vi "CSM - Read Config Cluster(Variant).vi"(4 "Write If not found?":bool, 5 "Section Name(\"\" as Default)":string, 7 "error in (no error)":errorcluster, 9 "Variant":variant) -> (1 "error out":errorcluster, 3 "Variant":variant)   [LabVIEW 2017, in "INI-Static-Variable-Support.lvlib"]
uses:
  INI-Static-Variable-Support.lvlib
  _fgv-oper.ctl
  fda69cd8-9796-4e90-9db0-f860da454eb2.vi
  global-csm-ini-db-change-flag.vi
  <userlib>/_NEVSTOP/Communicable State Machine(CSM)/addons/API-String-Arugments-Support/_Support/Data To API String Arguments.vi
  <userlib>/_NEVSTOP/Communicable State Machine(CSM)/addons/API-String-Arugments-Support/API String Arguments Support.lvlib
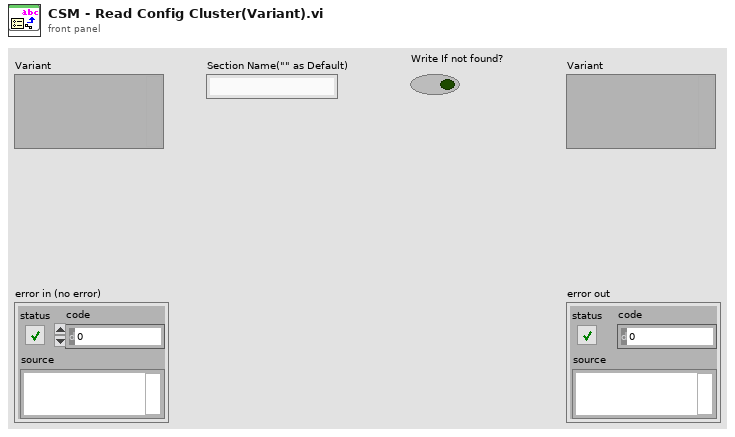
[diagram p1: front panel]
types:
  T1 = typedef "INI-Static-Variable-Support.lvlib/_fgv-oper.ctl" = enum16{"Read", "Write", "Sync"}
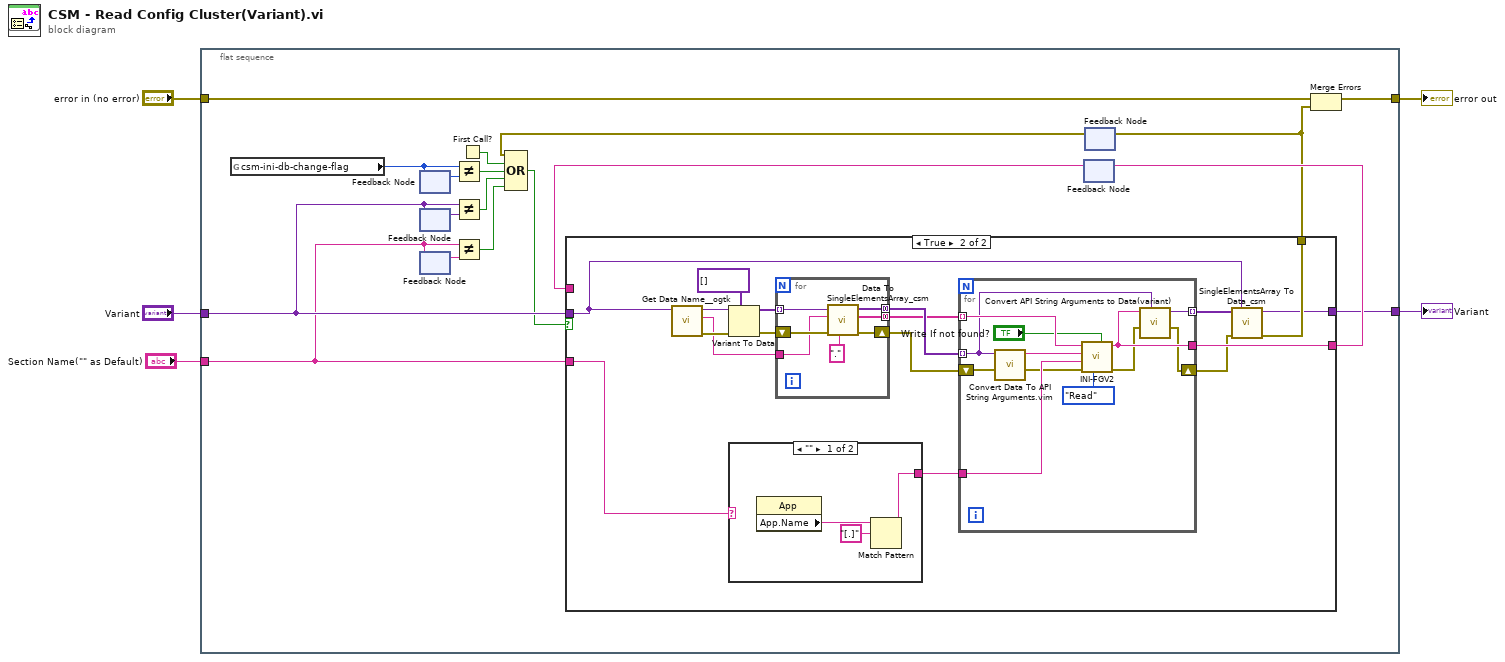
[diagram p0: block diagram]
diagram:
  n1 = flat-sequence {
    tunnel: [w23] -> w5
    tunnel: "error in (no error)" -> [w22]
    tunnel: "Variant" -> [w15]
    tunnel: "Section Name(\"\" as Default)" -> [w14]
    tunnel: [w6] -> w1
    frame #0 {
      n2 = global read "global-csm-ini-db-change-flag.vi" "csm-ini-db-change-flag"() -> (w21:u32)
      n3 = feedback #1() -> (w20:u32)  [unwired: 1 in]
      n4 = feedback-in #1(w21) -> ()
      n5 = feedback #2() -> (w17:variant)  [unwired: 1 in]
      n6 = feedback-in #2(w15) -> ()
      n7 = feedback #3() -> (w16:string)  [unwired: 1 in]
      n8 = feedback-in #3(w14) -> ()
      n9 = Not Equal?(x=w21, y=w20) -> (x != y?=w19:bool)
      n10 = Not Equal?(x=w15, y=w17) -> (x != y?=w13:bool)
      n11 = Not Equal?(x=w14, y=w16) -> (x != y?=w12:bool)
      n12 = First Call?() -> (First Call?: T/F=w18:bool)
      n13 = feedback #4() -> (w10:string)  [unwired: 1 in]
      n14 = feedback #5() -> (w8:errorcluster)  [unwired: 1 in]
      n15 = Compound Arithmetic op=OR(w8, w18, w19, w13, w12) -> (w7:bool)
      n16 = case shown="True" w7 {
        tunnel: [_ w35] -> w9
        tunnel: [w25 w42] -> w11
        tunnel: w15 -> [w24 w31]
        tunnel: w14 -> [_ w41]
        tunnel: w10 -> [w25 _]
        tunnel: [w24 w34] -> w6
        frame False {
        }
        frame True {
          n17 = call <userlib>:"Get Data Name__ogtk.vi"("Data"=w31) -> ("error out"=w27:errorcluster, "Data Name"=w26:string, "Data dup"=w28:variant)  [unwired: 8 in]
          n18 = Variant To Data(error in=w27, type=variant[] [] ("Array"), Variant=w28) -> (data=w30:variant[], error out=w29:errorcluster)
          n19 = case shown="\"\"" w41 {
            selector: w41 -> [_ w65]
            tunnel: [w62 w65] -> w40
            frame "" {
              n20 = property class="App"() -> ("App.Name"=w63:string)  [unwired: 2 in, 2 out]
              n21 = Match Pattern(string=w63, regular expression="[.]") -> (before substring=w62:string)  [unwired: 1 in, 3 out]
            }
            frame Default {
            }
          }
          n22 = for {
            tunnel: [w48] -> w39 mode=concatenating
            tunnel: [w47] -> w38 mode=concatenating
            tunnel: w30 -> [w45] mode=indexing
            shift-right: [w46] -> w33
            shift-left: w29 -> [w44]
            tunnel: w26 -> [w43]
            n23 = call <userlib>:"Data To SingleElementsArray_csm.vi"("Seperator(/)"=".", "error in (no error)"=w44, "parentUrl"=w43, "Cluster"=w45) -> ("error out"=w46:errorcluster, "Full NameList"=w47:string[], "DataElementArray"=w48:variant[])  [unwired: 5 in]
          }
          n24 = for {
            tunnel: w39 -> [w55] mode=indexing
            tunnel: w38 -> [w57] mode=indexing
            tunnel: w40 -> [w60]
            tunnel: [w56] -> w42
            shift-right: [w53] -> w36
            shift-left: w33 -> [w52]
            tunnel: [w51] -> w37 mode=indexing
            n25 = call "Convert Data To API String Arguments.vim"("error in (no error)"=w52, "data"=w55) -> ("error out"=w58:errorcluster, "String"=w59:string)  [unwired: 6 in]
            n26 = call "INI-FGV2.vi"("Write If not found?"="Write If not found?", "Enum"=_fgv-oper."Read", "error IN"=w58, ">> Section >>"=w60, ">> Default Value >>"=w59, ">> Variable Name >>"=w57) -> ("error out"=w54:errorcluster, "Value"=w56:string)  [unwired: 3 in, 1 out]
            n27 = call <userlib>:"Convert API String Arguments to Data(variant).vi"("Type"=w55, "error in (no error)"=w54, "String"=w56) -> ("error"=w53:errorcluster, "Data"=w51:variant)  [unwired: 7 in]
          }
          n28 = call <userlib>:"SingleElementsArray To Data_csm.vi"("Pototype"=w31, "error in (no error)"=w36, "DataElementArray"=w37) -> ("error out"=w35:errorcluster, "Cluster"=w34:variant)  [unwired: 7 in]
        }
      }
      n29 = feedback-in #4(w11) -> ()
      n30 = feedback-in #5(w9) -> ()
      n31 = Merge Errors(w22, w9) -> (w23:errorcluster)
    }
  }
  "error out" <- w5
  "Variant" <- w1
